vi "1Dto1DSearch.vi"(8 "Array 2":u64[](array[numeric]), 11 "Array 1":u64[](array[numeric])) -> (0 "UnMatching numbers":u64[](array[numeric]), 3 "Matching numbers":dbl[](array[numeric]) format="%#_1g")   [LabVIEW 2023]
panel:
  # "Търси съвпадение на всеки елемент от вторият масив в първият.\nАко има такива ги добавя в нов масив. Индексите на елементите\nследват хронологията на откриването им. Array2 съдържа ли се в Array1?"
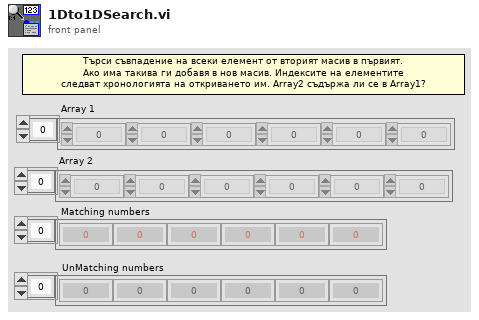
[diagram p1: front panel]
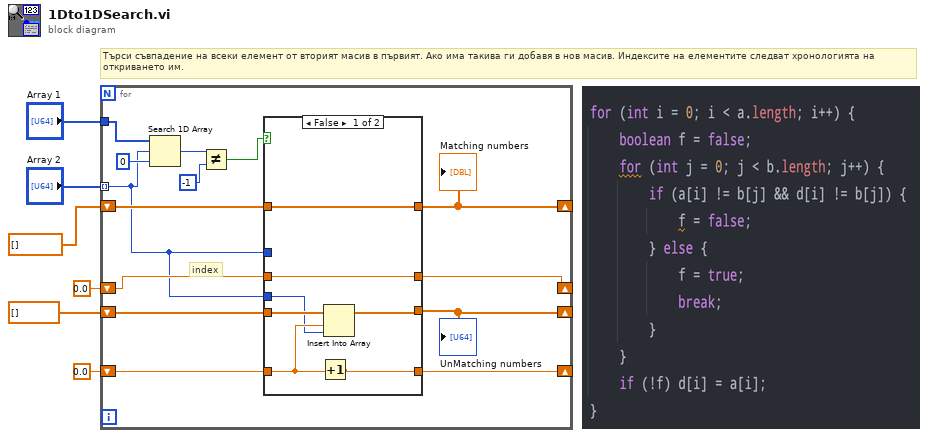
[diagram p0: block diagram]
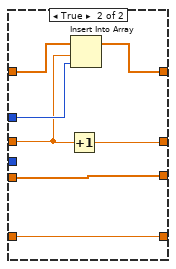
[diagram p2: hidden frame]
diagram:
  # "Търси съвпадение на всеки елемент от вторият масив в първият. Ако има такива ги добавя в нов масив. Индексите на елементите следват хронологията на откриването им."
  n1 = for {
    tunnel: "Array 1" -> [w20]
    tunnel: "Array 2" -> [w8] mode=indexing
    shift-right: [w16] -> _
    shift-left: dbl[] [] -> [w15]
    shift-right: [w13] -> _
    shift-left: 0.0 -> [w12]
    shift-right: [w7] -> _
    shift-left: 0.0 -> [w10]
    shift-right: [w11] -> _
    shift-left: dbl[] [] -> [w9]
    # "index"
    n2 = Search 1D Array(1D array=w20, element=w8, start index (0)=0) -> (index of element=w14:i32)
    n3 = Not Equal?(x=w14, y=-1) -> (x != y?=w17:bool)
    n4 = case shown="False" w17 {
      tunnel: w8 -> [_ w34]
      tunnel: w12 -> [w26 w31]
      tunnel: [w27 w33] -> w16
      tunnel: w15 -> [w27 w32]
      tunnel: [w26 w30] -> w13
      tunnel: [w25 w29] -> w11
      tunnel: [w24 w28] -> w7
      tunnel: w10 -> [w23 w28]
      tunnel: w9 -> [w22 w29]
      tunnel: w8 -> [w21 _]
      frame False {
        n5 = Increment(x=w23) -> (x+1=w24:dbl)
        n6 = Insert Into Array(array=w22, index=w23, new element=w21) -> (w25:dbl[])
      }
      frame True {
        n7 = Increment(x=w31) -> (x+1=w30:dbl)
        n8 = Insert Into Array "Insert Into Array"(array=w32, index=w31, new element=w34) -> (w33:dbl[])
      }
    }
    "Matching numbers" <- w16
    "UnMatching numbers" <- w11
  }
